vi "Encode Header and Payload.vi"(10 "Payload":string, 11 "Header":string) -> (2 "Encoded":string)   [LabVIEW 2017, in "JWT.lvlib"]
uses:
  JWT.lvlib
  lv-base64/Variant.ctl
  lv-base64/Base64.lvlib
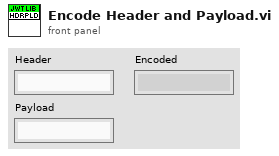
[diagram p1: front panel]
types:
  T1 = typedef "Base64.lvlib/Variant.ctl" = enum16{"Base64", "Base64-URL"}
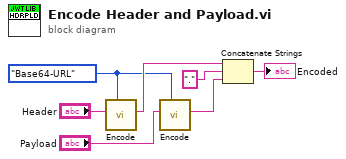
[diagram p0: block diagram]
diagram:
  w5 = Variant."Base64-URL" ("Variant (Base64)")
  n1 = call "Encode.vi"("Variant (Base64)"=w5, "string in (not encoded)"="Header") -> ("string out (base64-encoded)"=w6:string)  [unwired: 8 in, 1 out]
  n2 = call "Encode.vi"("Variant (Base64)"=w5, "string in (not encoded)"="Payload") -> ("string out (base64-encoded)"=w4:string)  [unwired: 8 in, 1 out]
  n3 = Concatenate Strings(w6, "." ("string"), w4) -> (→"Encoded":string)
